vi "Set Arm Position.vi"(0 "Button  States":cluster{"Lower":bool, "Middle":bool, "Top":bool}, 1 "Acquiring":bool, 2 "Right Stick Value":dbl, 3 "Low Eject":bool) -> (10 "Position out":dbl)   [LabVIEW 2015]
uses:
  Robot Values.vi
  <vilib>/ptbypt/NI_PtbyPt.lvlib
panel:
  in  "Top Angle":dbl=90.0 format="%#_13g"
  in  "Middle Angle":dbl=50.0 format="%#_13g"
  in  "Bottom Angle":dbl format="%#_13g"
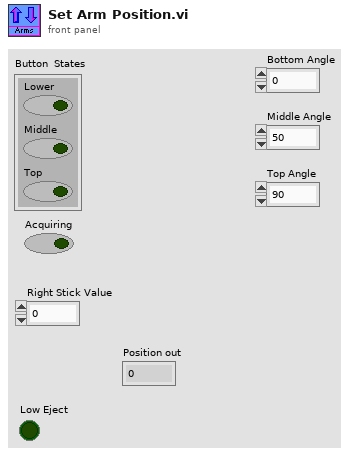
[diagram p1: front panel]
types:
  T1 = typedef "Robot Values.ctl" = cluster{"Drive Motors":cluster{"Left Motor Value":dbl, "Right Motor Value":dbl, "Left Motor Encoder":dbl, "Right Motor Encoder":dbl, "High/Low Gear":bool}, "Sensors":cluster{"Gyro Angle":dbl, "Photoeye":bool, "Ultrasonic Range":dbl, "Shooter Speed Encoder":dbl, "Accelerometer Value":dbl, "Flashlight":bool, "Target Distance":dbl, "Target X Value":dbl}, "Arms":cluster{"Desired Arm Position":dbl, "Left Arm Encoder":dbl, "Right Arm Encoder":dbl, "Left Arm Lower Limit":bool, "Right Arm Lower Limit":bool, "Initialize Arm Position?":bool}, "Acquisition and Scoring":cluster{"Acquiring?":bool, "Current Speed":dbl, "Setpoint Speed":dbl, "Prep Wheels":bool, "Shoot":bool, "Low Eject":bool}, "Hanging":cluster{"Pivot Arms":dbl, "PTO":bool, "Left Pivot Encoder":dbl, "Right Pivot Encoder":dbl, "Hanging Pin":bool}}
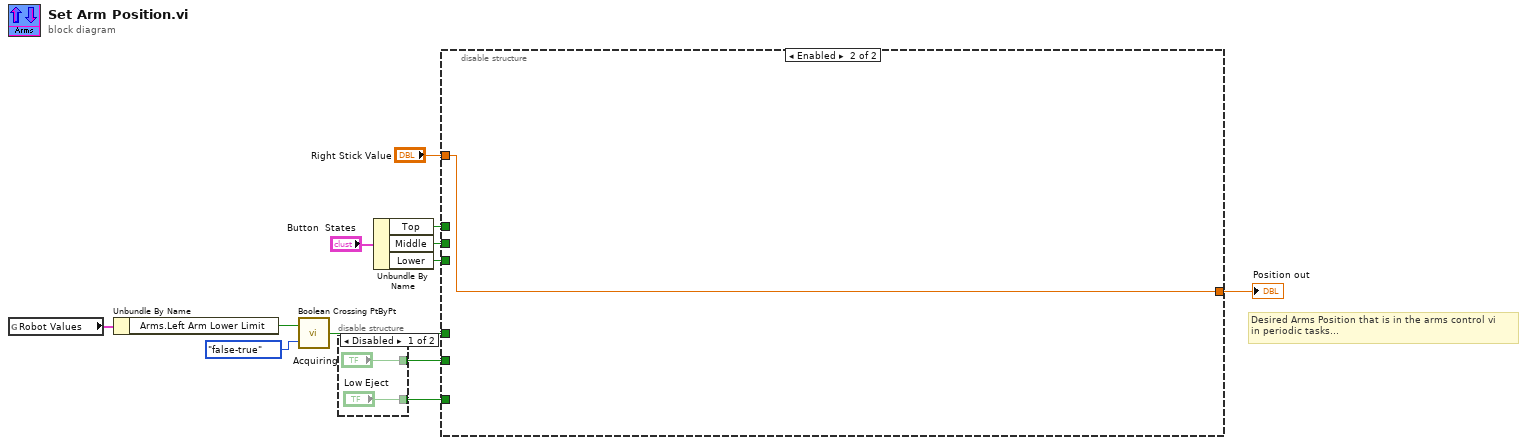
[diagram p0: block diagram]
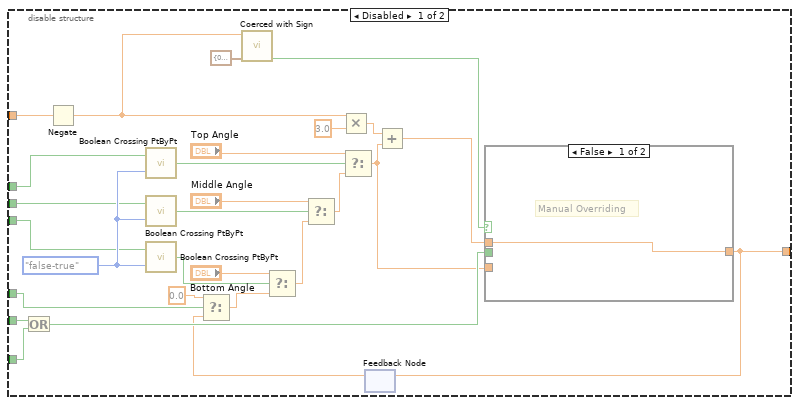
[diagram p3: hidden frame]
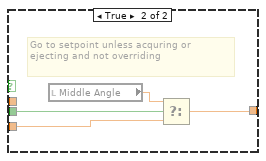
[diagram p4: hidden frame]
diagram:
  # "Desired Arms Position that is in the arms control vi\nin periodic tasks..."
  n1 = global read "Robot Values.vi" "Robot Values"() -> (w4:T1)
  n2 = Unbundle By Name(w4) -> ("Arms.Left Arm Lower Limit"=w3:bool)
  n3 = call <vilib>:"Boolean Crossing PtByPt.vi"("direction"=enum16{"either", "false-true", "true-false"}."false-true", "input"=w3) -> ("crossing"=w2:bool)  [unwired: 1 in]
  n4 = disable-structure shown="Disabled" {
    disable-tunnel: ["Acquiring" _] -> w8
    disable-tunnel: ["Low Eject" _] -> w7
    frame Disabled {
    }
    frame Enabled {
    }
  }
  n5 = Unbundle By Name("Button  States") -> ("Top"=w11:bool, "Middle"=w10:bool, "Lower"=w9:bool)
  n6 = disable-structure shown="Enabled" {
    disable-tunnel: w11 -> [w31 _]
    disable-tunnel: w10 -> [w30 _]
    disable-tunnel: w9 -> [w29 _]
    disable-tunnel: w8 -> [w28 _]
    disable-tunnel: w7 -> [w26 _]
    disable-tunnel: "Right Stick Value" -> [w25 w48]
    disable-tunnel: [w20 w48] -> w5
    disable-tunnel: w2 -> [w18 _]
    frame Disabled {
      w37 = enum16{"either", "false-true", "true-false"}."false-true" ("direction")
      n7 = Or(x=w28, y=w26) -> (x .or. y?=w27:bool)
      n8 = Negate(x=w25) -> (-x=w19:dbl)
      n9 = call <vilib>:"Boolean Crossing PtByPt.vi"("direction"=w37, "input"=w31) -> ("crossing"=w38:bool)  [unwired: 1 in]
      n10 = call <vilib>:"Boolean Crossing PtByPt.vi"("direction"=w37, "input"=w30) -> ("crossing"=w40:bool)  [unwired: 1 in]
      n11 = call <vilib>:"Boolean Crossing PtByPt.vi"("direction"=w37, "input"=w29) -> ("crossing"=w42:bool)  [unwired: 1 in]
      n12 = call "Coerced with Sign.vi"("Input"=w19, "Limits"=cluster{"\"Upper\"":dbl, "\"Lower\"":dbl} {"\"Upper\""=0.2, "\"Lower\""=-0.2}) -> ("In Range?"=w23:bool)  [unwired: 7 in, 1 out]
      n13 = Multiply(x=w19, y=3.0) -> (x*y=w35:dbl)
      n14 = feedback #1() -> (w16:dbl)  [unwired: 1 in]
      n15 = Select(t=0.0, s=w18, f=w16) -> (s? t:f=w15:dbl)
      n16 = Select(t="Bottom Angle", s=w42, f=w15) -> (s? t:f=w41:dbl)
      n17 = Select(t="Middle Angle", s=w40, f=w41) -> (s? t:f=w39:dbl)
      n18 = Select(t="Top Angle", s=w38, f=w39) -> (s? t:f=w21:dbl)
      n19 = Add(x=w35, y=w21) -> (x+y=w22:dbl)
      n20 = case shown="False" w23 {
        tunnel: w27 -> [_ w45]
        tunnel: [w43 w44] -> w20
        tunnel: w22 -> [w43 _]
        tunnel: w21 -> [_ w47]
        frame False {
          # "Manual Overriding"
        }
        frame True {
          # "Go to setpoint unless acquring or ejecting and not overriding"
          n21 = local read "Middle Angle"() -> (w46:dbl)
          n22 = Select(t=w46, s=w45, f=w47) -> (s? t:f=w44:dbl)
        }
      }
      n23 = feedback-in #1(w20) -> ()
    }
    frame Enabled {
    }
  }
  "Position out" <- w5
